vi "Destroy.vi"(8 "error in (no error)":errorcluster, 11 "Gluing Procedure in":refnum<class "Gluing Procedure.lvclass">) -> (0 "error out":errorcluster)   [LabVIEW 2011, in "Gluing Procedure.lvclass"]
uses:
  Gluing Procedure.lvclass
  Gluing Procedure.lvclass/Gluing Procedure.ctl
  Shared Components/Gantry Class/Gantry Class.lvclass
  Shared Components/Config Manager Class/Config Manager Class.lvclass
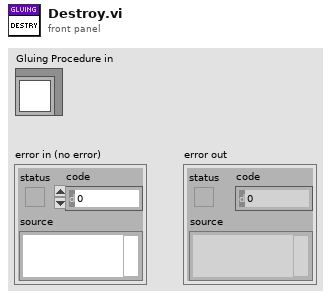
[diagram p1: front panel]
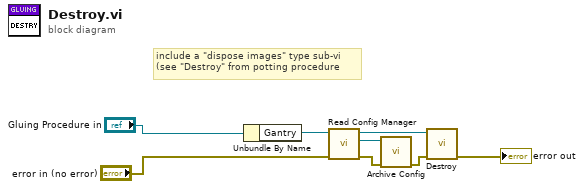
[diagram p0: block diagram]
diagram:
  # "include a \"dispose images\" type sub-vi\n(see \"Destroy\" from potting procedure"
  n1 = Unbundle By Name("Gluing Procedure in") -> ("Gantry"=w8:refnum<class "Gantry Class.lvclass">)
  n2 = call-dynamic "Read Config Manager.vi"("error in"="error in (no error)", "Gantry in"=w8) -> ("error out"=w6:errorcluster, "Config Manager"=w7:refnum<class "Config Manager Class.lvclass">, "Gantry out"=w5:refnum<class "Gantry Class.lvclass">)  [unwired: 7 in]
  n3 = call "Archive Config.vi"("error in"=w6, "Config Manager in"=w7) -> ("error out"=w4:errorcluster)  [unwired: 8 in, 1 out]
  n4 = call "Destroy.vi"("error in"=w4, "Gantry Class in"=w5) -> ("error out"=→"error out":errorcluster)  [unwired: 9 in]
